vi "Add Data Point.vi"(7 "row index (0)":i32, 8 "pixel position":cluster{"X":i32, "Y":i32}, 9 "DrawAreaSize":T1={"Width"=100, "Height"=100}, 10 "draw options":T2={"Background Color"=16777215, "Grid Color"=13816530, "Angle Units"=enum."Degrees", "Draw Solid Background"=TRUE, "Draw Grid"=TRUE, "Grid Spacing"=0.25, "AutoScale"=FALSE, "Fit to Radius"=1.0, "data row options"=[]}, 11 "data in":T5) -> (3 "data out":T5)   [LabVIEW 2017, in "NI_Robotics_2D Rangefinder Picture.lvlib"]
uses:
  <vilib>/robotics/Controls/2D Rangefinder/2D Rangefinder Picture/NI_Robotics_2D Rangefinder Picture.lvlib
  <vilib>/robotics/Controls/2D Rangefinder/2D Rangefinder Picture/Rangefinder Data.ctl
  <vilib>/robotics/Controls/2D Rangefinder/2D Rangefinder Picture/Draw Options.ctl
  <vilib>/robotics/Controls/Utilities/Angle Units.ctl
  <vilib>/robotics/Controls/2D Rangefinder/2D Rangefinder Picture/Data Row Options.ctl
  <vilib>/Utility/miscctls.llb/LVBoundsTypeDef.ctl
  <vilib>/Utility/AngleManip/Radians to Degrees (Scalar DBL).vi
  <vilib>/Utility/AngleManip/Degrees to Radians.vi
  <vilib>/Utility/AngleManip/Degrees to Radians (Array DBL).vi
  <vilib>/Utility/AngleManip/NI_AngleManipulation.lvlib
  <vilib>/robotics/Controls/Utilities/NI_Robotics_Control Utilities.lvlib
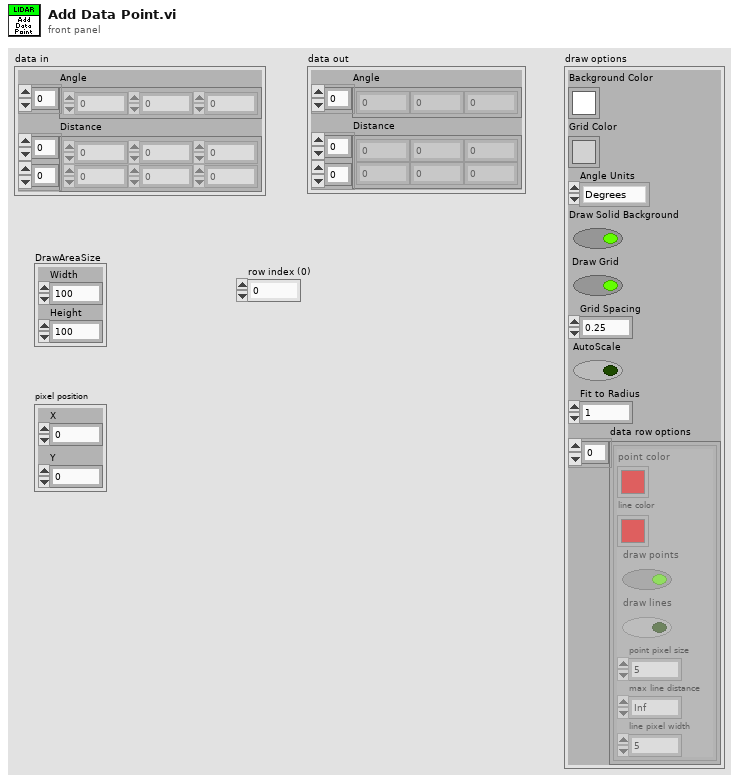
[diagram p1: front panel]
types:
  T1 = typedef "LVBoundsTypeDef.ctl" = cluster{"Width":u32, "Height":u32}
  T2 = typedef "NI_Robotics_2D Rangefinder Picture.lvlib/Draw Options.ctl" = cluster{"Background Color":u32, "Grid Color":u32, "Angle Units":T3, "Draw Solid Background":bool, "Draw Grid":bool, "Grid Spacing":dbl, "AutoScale":bool, "Fit to Radius":dbl, "data row options":T4[]}
  T3 = typedef "NI_Robotics_Control Utilities.lvlib/Angle Units.ctl" = enum16{"Radians", "Degrees"}
  T4 = typedef "NI_Robotics_2D Rangefinder Picture.lvlib/Data Row Options.ctl" = cluster{"point color":u32, "line color":u32, "draw points":bool, "draw lines":bool, "point pixel size":u16, "max line distance":dbl, "line pixel width":u16}
  T5 = typedef "NI_Robotics_2D Rangefinder Picture.lvlib/Rangefinder Data.ctl" = cluster{"Angle":dbl[], "Distance":dbl[][]}
  T6 = typedef "NI_Robotics_2D Rangefinder Picture.lvlib/Cartesian Data.ctl" = cluster{"xy points":cluster{"xy set":cluster{"x":dbl, "y":dbl}[], "distance set":dbl[]}[], "max radius":dbl}
  T7 = typedef "NI_Robotics_2D Rangefinder Picture.lvlib/Scaling Info.ctl" = cluster{"pixels per unit":dbl, "fit radius (units)":dbl, "center point (pixels)":cluster{"x":i16, "y":i16}}
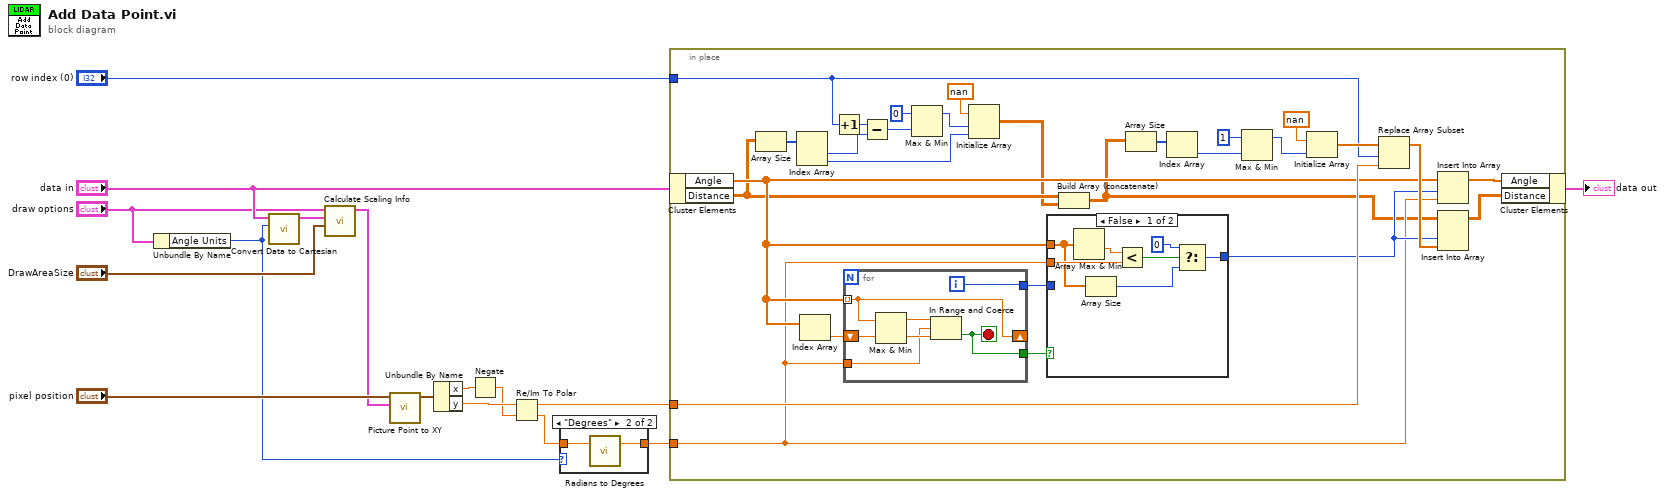
[diagram p0: block diagram]
diagram:
  n1 = Unbundle By Name("draw options") -> ("Angle Units"=w1:T3)
  n2 = call <vilib>:"Convert Data to Cartesian.vi"("angle units"=w1, "data"="data in") -> ("cartesian data"=w16:T6)  [unwired: 9 in]
  n3 = call <vilib>:"Calculate Scaling Info.vi"("DrawAreaSize"="DrawAreaSize", "cartesian data"=w16, "draw options in"="draw options") -> ("scaling info"=w13:T7)  [unwired: 8 in]
  n4 = call <vilib>:"Picture Point to XY.vi"("scaling info"=w13, "xy point (pixels)"="pixel position") -> ("xy point (units)"=w10:cluster{"x":dbl, "y":dbl})  [unwired: 9 in]
  n5 = Unbundle By Name(w10) -> ("x"=w9:dbl, "y"=w8:dbl)
  n6 = Negate(x=w9) -> (-x=w7:dbl)
  n7 = Re/Im To Polar(2:w7, 3:w8) -> (0:w5:dbl, 1:w4:dbl)
  n8 = case shown="\"Degrees\"" w1 {
    tunnel: w5 -> [w17 w19]
    tunnel: [w17 w18] -> w3
    frame "Radians", Default {
    }
    frame "Degrees" {
      n9 = call-poly <vilib>:"Radians to Degrees.vi"("angle (rad)"=w19) -> ("angle (deg)"=w18:dbl)  [unwired: 2 in]
    }
  }
  n10 = in-place {
    in-place-border: w4 -> [w41]
    in-place-border: w3 -> [w33]
    in-place-border: "row index (0)" -> [w32]
    n11 = in-place-cluster #1("data in") -> ("Angle"=w34:dbl[], "Distance"=w25:dbl[][])
    n12 = Array Size(array=w25) -> (size(s)=w45:i32[])
    n13 = Index Array(array=w45) -> (element #1=w21:i32, element #2=w26:i32)  [unwired: 2 in]
    n14 = Index Array(array=w34) -> (element=w38:dbl)  [unwired: 1 in]
    n15 = Increment(x=w32) -> (x+1=w31:i32)
    n16 = for {
      tunnel: w34 -> [w61] mode=indexing
      shift-right: [w61] -> _
      shift-left: w38 -> [w62]
      tunnel: w33 -> [w58]
      tunnel: [w57] -> w36
      tunnel: [w56] -> w37
      i -> [w57]
      stop <- w56 stop-if-true
      n17 = Max & Min(x=w61, y=w62) -> (max(x,y)=w60:dbl, min(x,y)=w59:dbl)
      n18 = In Range and Coerce(upper limit=w60, x=w58, lower limit=w59) -> (In Range?=w56:bool)  [unwired: 1 out]
    }
    n19 = Subtract(x=w31, y=w21) -> (x-y=w29:i32)
    n20 = Max & Min(x=0, y=w29) -> (max(x,y)=w27:i32)  [unwired: 1 out]
    n21 = Initialize Array(nan ("element"), w27, w26) -> (w24:dbl[][])
    n22 = case shown="False" w37 {
      tunnel: w36 -> [_ w55]
      tunnel: [w48 w55] -> w35
      tunnel: w34 -> [w52 _]
      tunnel: w33 -> [w53 _]
      frame False {
        n23 = Array Max & Min(array=w52) -> (min value=w54:dbl)  [unwired: 3 out]
        n24 = Array Size(array=w52) -> (size(s)=w49:i32)
        n25 = Less?(x=w54, y=w53) -> (x < y?=w50:bool)
        n26 = Select(t=0, s=w50, f=w49) -> (s? t:f=w48:i32)
      }
      frame True {
      }
    }
    n27 = Build Array (concatenate)(w25, w24) -> (w22:dbl[][])
    n28 = Array Size(array=w22) -> (size(s)=w23:i32[])
    n29 = Index Array(array=w23) -> (element=w20:i32)  [unwired: 1 in]
    n30 = Max & Min(x=1, y=w20) -> (max(x,y)=w39:i32)  [unwired: 1 out]
    n31 = Initialize Array(nan ("element"), w39) -> (w43:dbl[])
    n32 = Replace Array Subset(array=w43, new element=w41, index=w32) -> (w42:dbl[])
    n33 = Insert Into Array(array=w34, index=w35, new element=w33) -> (w47:dbl[])
    n34 = Insert Into Array(array=w22, index (col)=w35, new element=w42) -> (w46:dbl[][])  [unwired: 1 in]
    n35 = in-place-cluster #1("Angle"=w47, "Distance"=w46) -> (→"data out":T5)
  }
